vi "Reports.Results TE to Test Result Pre JSON V2.vi"(4 "File Data Objs":T1[](array[typedef]), 5 "Test Result In":T10={"#attributes"={"Version"="MTE_1.0.0"}, "Station"={"Name"="", "PN"="", "SN"="", "Rev"="", "PC Name"="", "Location"="", "HW_Config"={"HW_Item"=[]}, "SW_Config"={"SW_Item"=[]}}, "Test Run"={"Operator"="", "Start Time"=timestamp(0 s since 1904-01-01), "Duration(s)"=0.0, "Mode"="", "Comment"="", "ProcessStep"=""}, "Test Sequence"={"Name"="", "Config"={"Config_Item"=[]}}, "UUTs"={"UUT"=[]}} {"UUTs"."UUT"."Measurements"."Measurement"."Status" items=["LOG", "PASS", "FAIL", "ERROR"]}) -> (1 "Test Result V2":T2={"Type"="Test Data", "Version"="1.0.0", "TestEvent"={"ProcessStep"="", "StartTime"="", "EndTime"="", "Mode"="", "Operator"="", "Comment"="", "Result"={"State"="", "Code"=0, "Desc"="", "Details"=""}}, "UUTInfo"={"Product"="", "Description"="", "PN"="", "SN"="", "LotNumber"="", "DateCode"="", "AltID"="", "Revision"="", "Properties"=[]}, "Station"={"Name"="", "Location"="", "ConfigID"="", "PCName"="", "Slot"=""}, "TestSequence"={"Name"="", "Setup"=[]}, "ResultData"=[], "DataObjs"=[]})   [LabVIEW 2018]
uses:
  Results/Result XML/TestResult.FullResultData.ctl
  Results/Result XML/TestResult.Station Info.ctl
  Results/Result XML/TestResult.HW Item.ctl
  Results/Result XML/TestResult.SW Item.ctl
  Results/Result XML/TestResult.Test Run Info.ctl
  Results/Result XML/TestResult.Test Info.ctl
  Results/Result XML/TestResult.UUT Result.ctl
  Results/Result XML/TestResult.Symptom.ctl
  Results/Result XML/TestResult.Symptom.State.ctl
  Results/Result.Measurement Item.ctl
  Results/Result.Measurement and Attribute Item Status.ctl
  Results/Result XML/TestResult.UUTInfo.ctl
  Report.Result Data JSON V2.0.0.ctl
  Report.Result Test Event.ctl
  Report.Result State.ctl
  Report.Result UUTInfo.ctl
  Report.Result Test Station.ctl
  Report.Result Test Sequence.ctl
  Report.Result Measurement JSON Safe.ctl
  Report.Result DataObject.ctl
  Report.Result FileDataObject.ctl
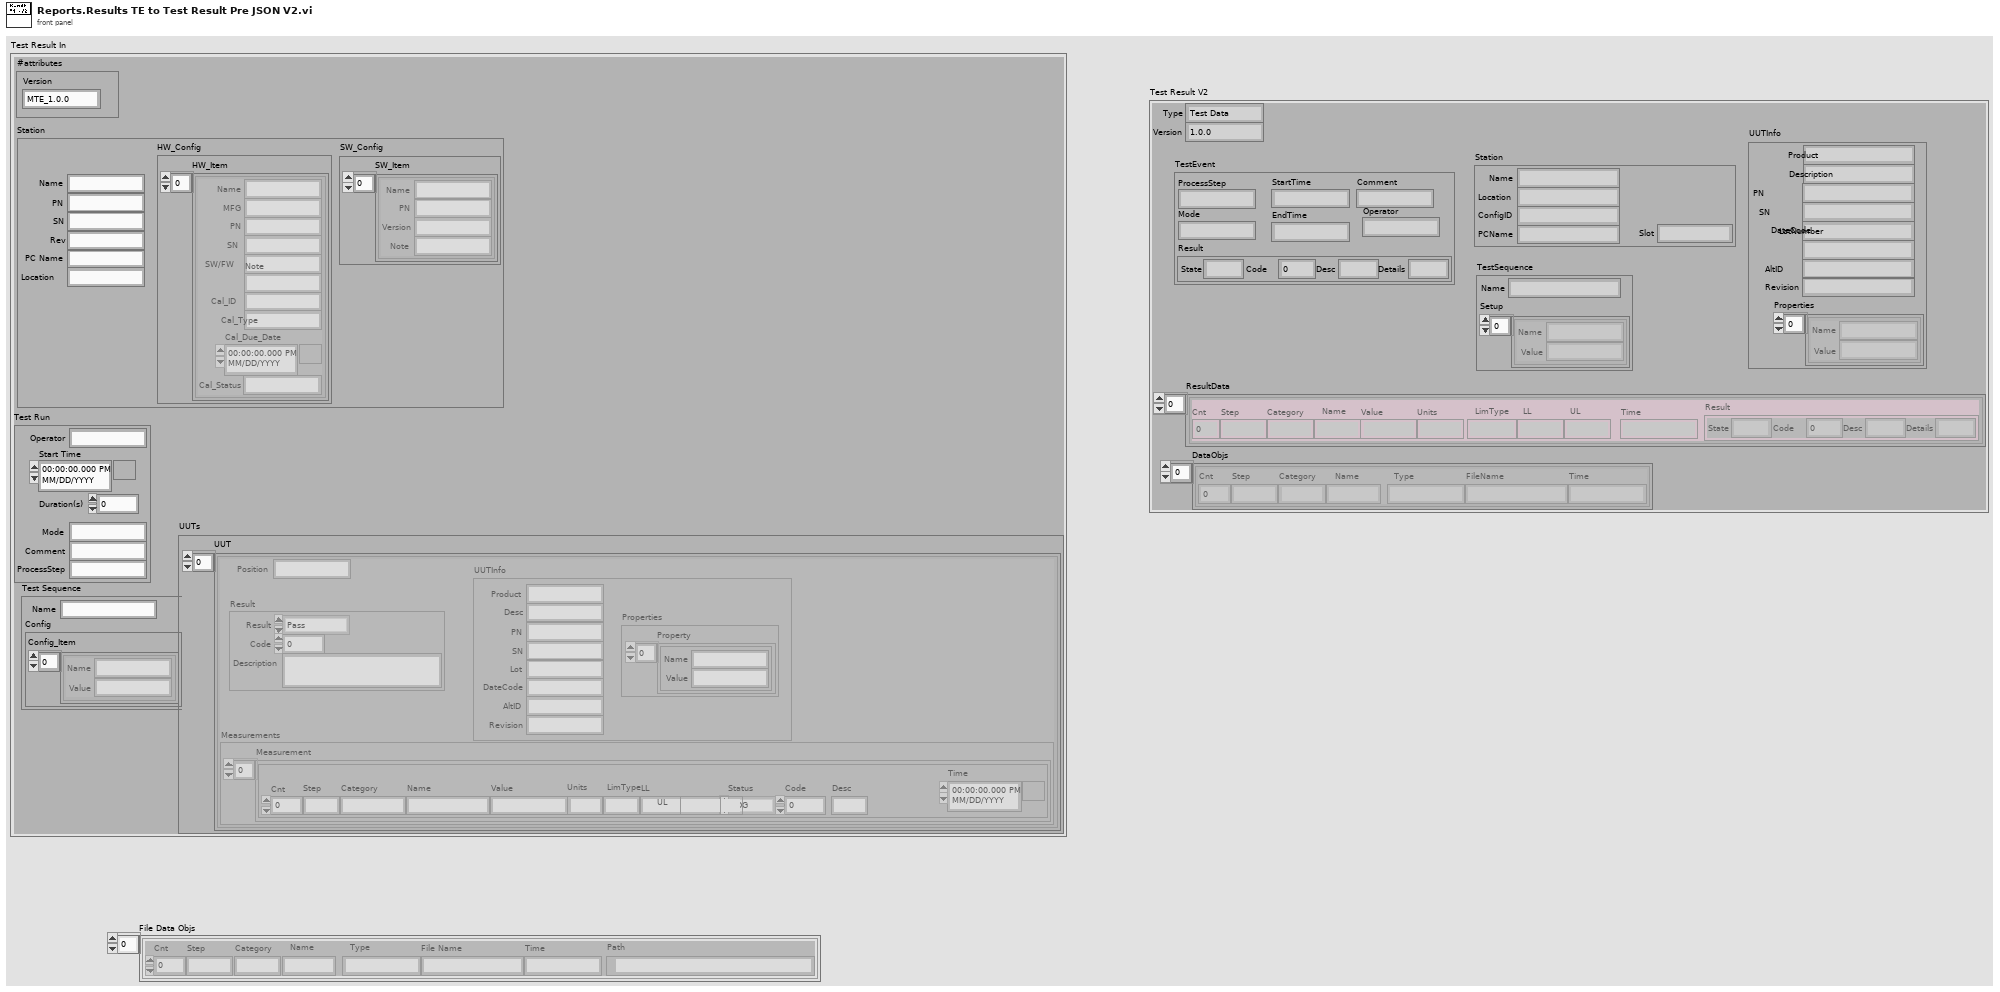
[diagram p1: front panel]
types:
  T1 = typedef "Report.Result FileDataObject.ctl" = cluster{"Cnt":i32, "Step":string, "Category":string, "Name":string, "Type":string, "File Name":string, "Time":string, "Path":path}
  T2 = typedef "Report.Result Data JSON V2.0.0.ctl" = cluster{"Type":string, "Version":string, "TestEvent":T3, "UUTInfo":T5, "Station":T6, "TestSequence":T7, "ResultData":T8[], "DataObjs":T9[]}
  T3 = typedef "Report.Result Test Event.ctl" = cluster{"ProcessStep":string, "StartTime":string, "EndTime":string, "Mode":string, "Operator":string, "Comment":string, "Result":T4}
  T4 = typedef "Report.Result State.ctl" = cluster{"State":string, "Code":i32, "Desc":string, "Details":string}
  T5 = typedef "Report.Result UUTInfo.ctl" = cluster{"Product":string, "Description":string, "PN":string, "SN":string, "LotNumber":string, "DateCode":string, "AltID":string, "Revision":string, "Properties":cluster{"Name":string, "Value":string}[]}
  T6 = typedef "Report.Result Test Station.ctl" = cluster{"Name":string, "Location":string, "ConfigID":string, "PCName":string, "Slot":string}
  T7 = typedef "Report.Result Test Sequence.ctl" = cluster{"Name":string, "Setup":cluster{"Name":string, "Value":string}[]}
  T8 = typedef "Report.Result Measurement JSON Safe.ctl" = cluster{"Cnt":i32, "Step":string, "Category":string, "Name":string, "Value":string, "Units":string, "LimType":string, "LL":string, "UL":string, "Time":string, "Result":T4}
  T9 = typedef "Report.Result DataObject.ctl" = cluster{"Cnt":i32, "Step":string, "Category":string, "Name":string, "Type":string, "FileName":string, "Time":string}
  T10 = typedef "TestResult.FullResultData.ctl" = cluster{"#attributes":cluster{"Version":string}, "Station":T11, "Test Run":T14, "Test Sequence":T15, "UUTs":cluster{"UUT":T16[]}}
  T11 = typedef "TestResult.Station Info.ctl" = cluster{"Name":string, "PN":string, "SN":string, "Rev":string, "PC Name":string, "Location":string, "HW_Config":cluster{"HW_Item":T12[]}, "SW_Config":cluster{"SW_Item":T13[]}}
  T12 = typedef "TestResult.HW Item.ctl" = cluster{"Name":string, "MFG":string, "PN":string, "SN":string, "SW/FW":string, "Note":string, "Cal_ID":string, "Cal_Type":string, "Cal_Due_Date":timestamp, "Cal_Status":string}
  T13 = typedef "TestResult.SW Item.ctl" = cluster{"Name":string, "PN":string, "Version":string, "Note":string}
  T14 = typedef "TestResult.Test Run Info.ctl" = cluster{"Operator":string, "Start Time":timestamp, "Duration(s)":dbl, "Mode":string, "Comment":string, "ProcessStep":string}
  T15 = typedef "TestResult.Test Info.ctl" = cluster{"Name":string, "Config":cluster{"Config_Item":cluster{"Name":string, "Value":string}[]}}
  T16 = typedef "TestResult.UUT Result.ctl" = cluster{"Position":string, "Result":T17, "Measurements":cluster{"Measurement":T19[]}, "UUTInfo":T21}
  T17 = typedef "TestResult.Symptom.ctl" = cluster{"Result":T18, "Code":i32, "Description":string}
  T18 = typedef "TestResult.Symptom.State.ctl" = enum16{"Pass", "Fail", "Error", "Aborted", "Completed", "Logged"}
  T19 = typedef "Result.Measurement Item.ctl" = cluster{"Cnt":i32, "Step":string, "Category":string, "Name":string, "Value":string, "Units":string, "LimType":string, "LL":string, "UL":string, "Status":T20, "Code":i32, "Desc":string, "Time":timestamp}
  T20 = typedef "Result.Measurement and Attribute Item Status.ctl" = i32
  T21 = typedef "TestResult.UUTInfo.ctl" = cluster{"Product":string, "Desc":string, "PN":string, "SN":string, "Lot":string, "DateCode":string, "AltID":string, "Revision":string, "Properties":cluster{"Property":cluster{"Name":string, "Value":string}[]}}
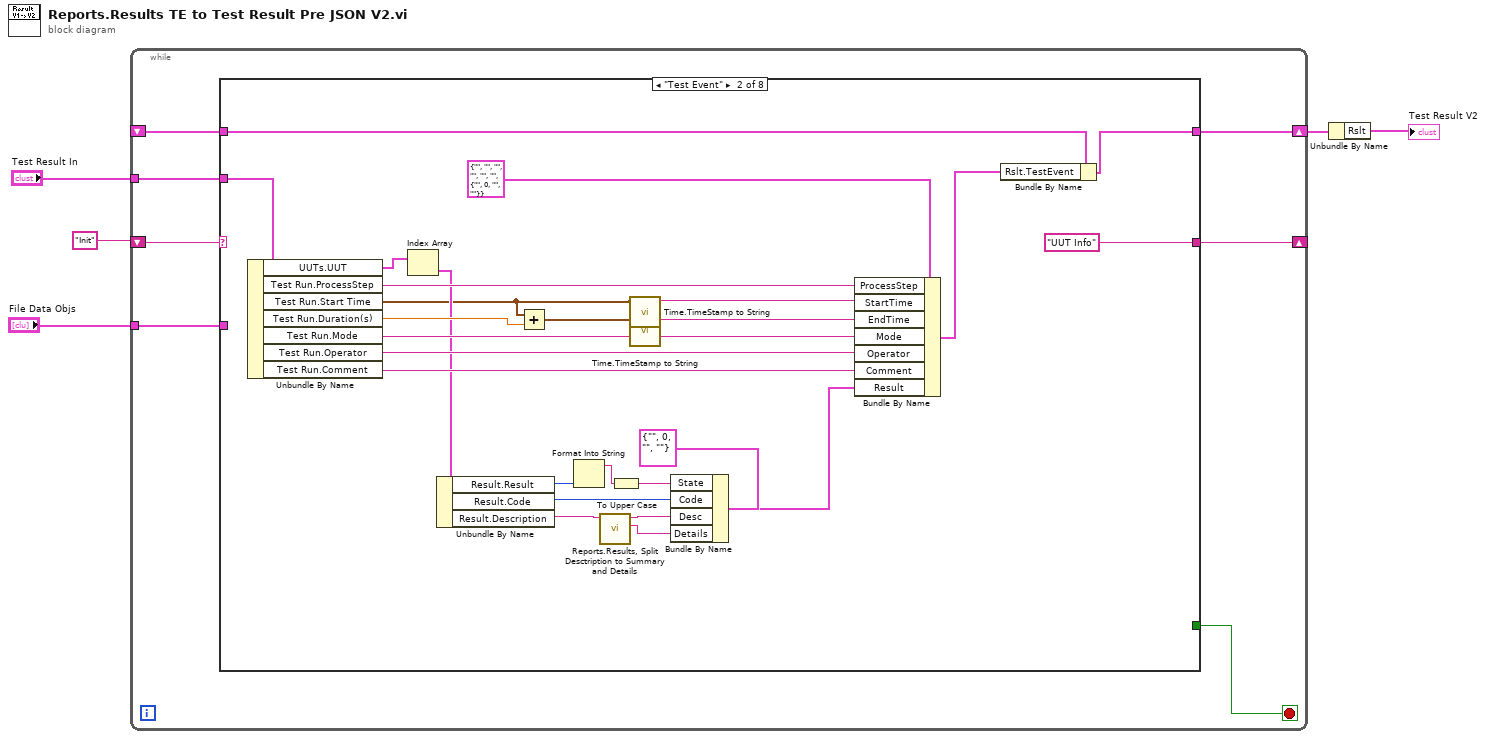
[diagram p0: block diagram]
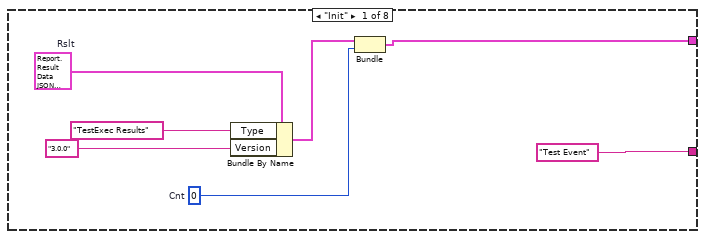
[diagram p2: hidden frame]
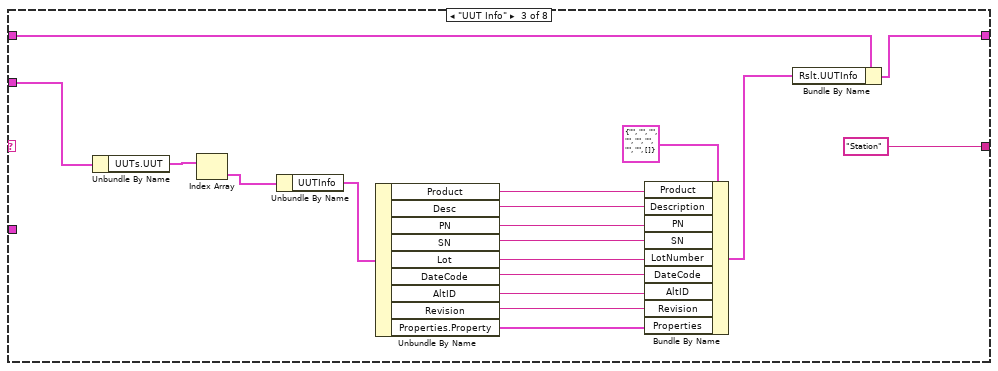
[diagram p3: hidden frame]
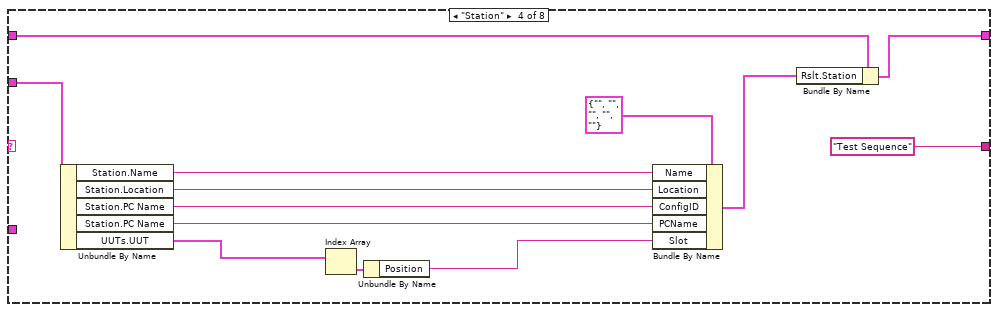
[diagram p4: hidden frame]
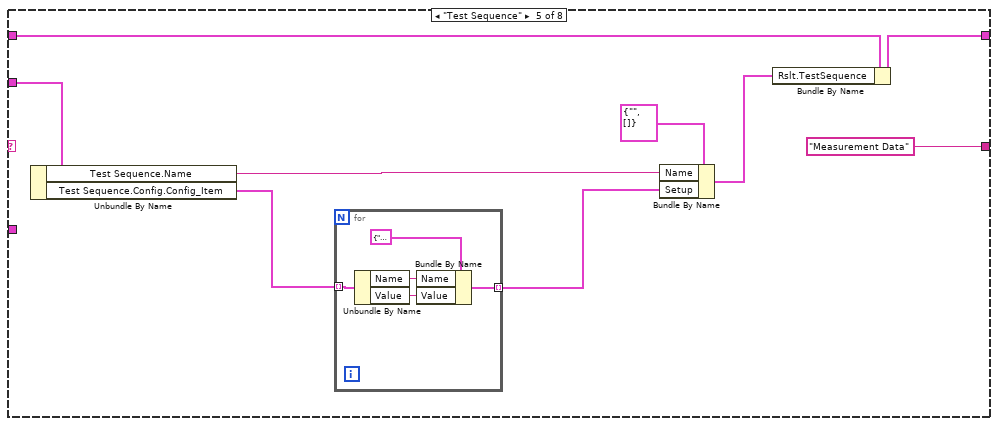
[diagram p5: hidden frame]
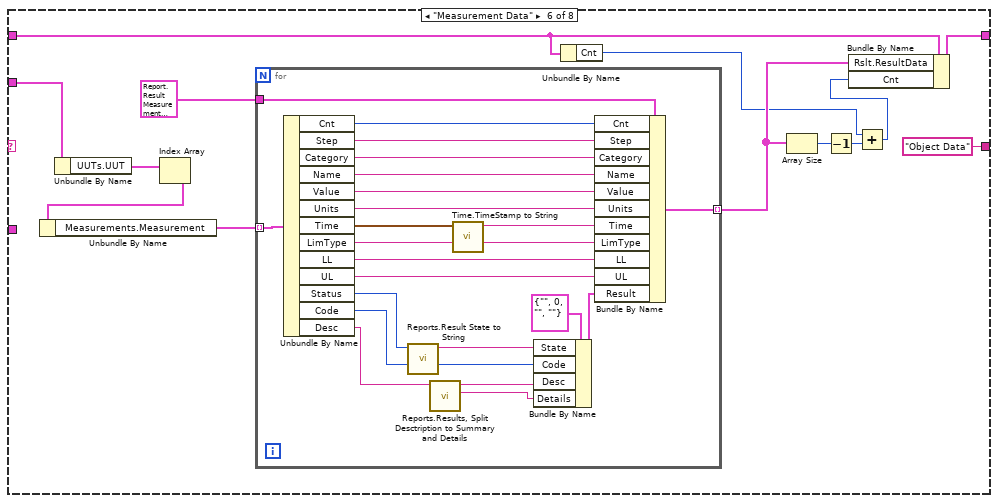
[diagram p6: hidden frame]
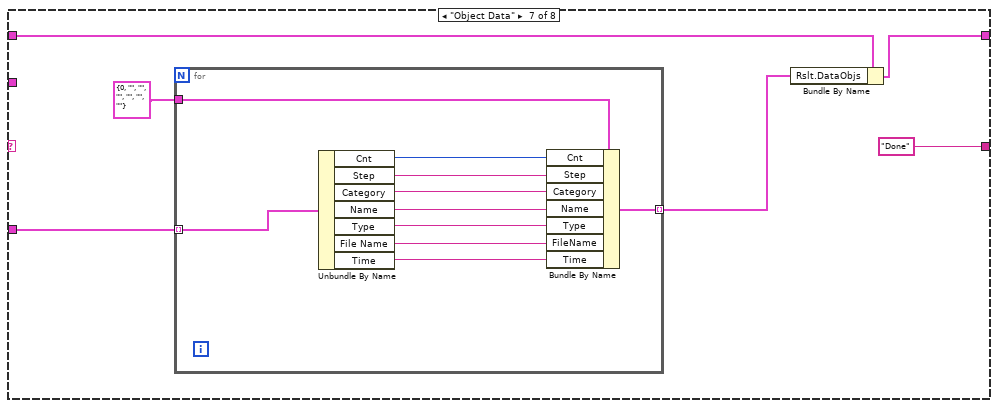
[diagram p7: hidden frame]
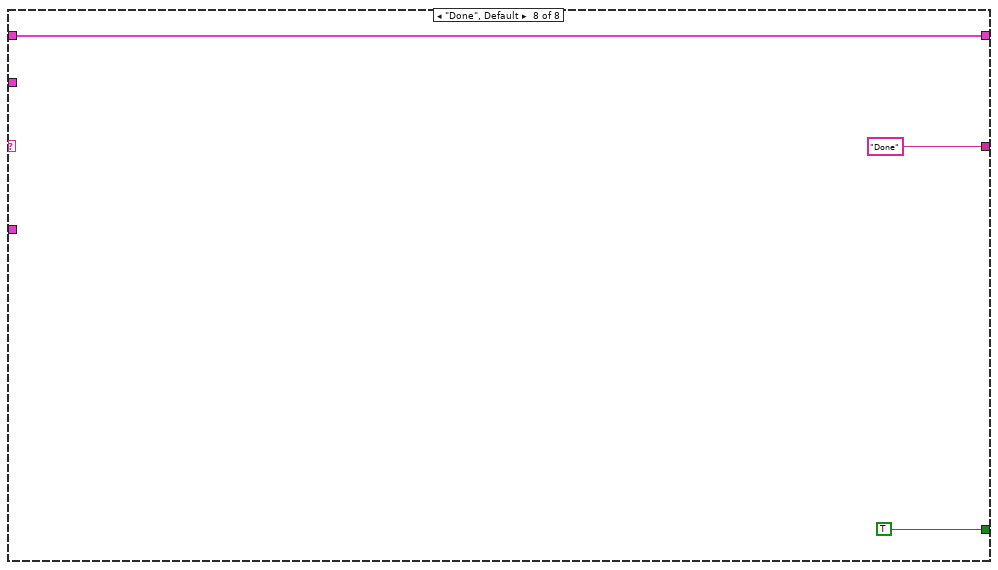
[diagram p8: hidden frame]
diagram:
  n1 = while {
    tunnel: "Test Result In" -> [w12]
    shift-right: [w10] -> w2
    shift-left: _ -> [w11]
    shift-right: [w7] -> _
    shift-left: "Init" -> [w8]
    tunnel: "File Data Objs" -> [w6]
    stop <- w9 stop-if-true
    n2 = case shown="\"Test Event\"" w8 {
      tunnel: w12 -> [_ w39 w59 w72 w81 w102 _ _]
      tunnel: w11 -> [_ w45 w63 w76 w85 w93 w126 w144]
      tunnel: [w14 w44 w62 w75 w84 w103 w131 w144] -> w10
      tunnel: [_ _ _ _ _ _ _ TRUE] -> w9
      tunnel: ["Test Event" ("Version") "UUT Info" ("Version") "Station" ("Version") "Test Sequence" ("Version") "Measurement Data" ("Version") "Object Data" ("Version") "Done" ("Version") "Done"] -> w7
      tunnel: w6 -> [_ _ _ _ _ _ w127 _]
      frame "Init" {
        w13 = 0  # Cnt
        w17 = T2 {"Type"="Test Data", "Version"="1.0.0", "TestEvent"={"ProcessStep"="", "StartTime"="", "EndTime"="", "Mode"="", "Operator"="", "Comment"="", "Result"={"State"="", "Code"=0, "Desc"="", "Details"=""}}, "UUTInfo"={"Product"="", "Description"="", "PN"="", "SN"="", "LotNumber"="", "DateCode"="", "AltID"="", "Revision"="", "Properties"=[]}, "Station"={"Name"="", "Location"="", "ConfigID"="", "PCName"="", "Slot"=""}, "TestSequence"={"Name"="", "Setup"=[]}, "ResultData"=[], "DataObjs"=[]}  # Rslt
        n3 = Bundle By Name(cluster=w17, "Type"="TestExec Results", "Version"="3.0.0") -> (w15:T2)
        n4 = Bundle("Rslt"=w15, "Cnt"=w13) -> (w14:cluster{"Rslt":T2, "Cnt":i32})  [unwired: 1 in]
      }
      frame "Test Event" {
        n5 = Unbundle By Name(w39) -> ("UUTs.UUT"=w38:T16[], "Test Run.ProcessStep"=w37:string, "Test Run.Start Time"=w27:timestamp, "Test Run.Duration(s)"=w35:dbl, "Test Run.Mode"=w36:string, "Test Run.Operator"=w34:string, "Test Run.Comment"=w33:string)
        n6 = Index Array(array=w38) -> (element=w32:T16)  [unwired: 1 in]
        n7 = Unbundle By Name(w32) -> ("Result.Result"=w30:T18, "Result.Code"=w31:i32, "Result.Description"=w22:string)
        n8 = Add(x=w27, y=w35) -> (x+y=w28:timestamp)
        n9 = Format Into String(w30) -> (resulting string=w23:string)  [unwired: 3 in, 1 out]
        n10 = call "Reports.Results, Split Desctription to Summary and Details.vi"("Description"=w22) -> ("Details"=w21:string, "Summary Description"=w20:string)  [unwired: 9 in]
        n11 = To Upper Case(1:w23) -> (0:w24:string)
        n12 = call "Time.TimeStamp to String.vi"("Time Stamp in"=w27) -> ("Time String Out"=w26:string)  [unwired: 10 in]
        n13 = call "Time.TimeStamp to String.vi"("Time Stamp in"=w28) -> ("Time String Out"=w25:string)  [unwired: 10 in]
        n14 = Bundle By Name(cluster=T4 {"State"="", "Code"=0, "Desc"="", "Details"=""} ("Result"), "State"=w24, "Code"=w31, "Desc"=w20, "Details"=w21) -> (w40:T4)
        n15 = Bundle By Name(cluster=T3 {"ProcessStep"="", "StartTime"="", "EndTime"="", "Mode"="", "Operator"="", "Comment"="", "Result"={"State"="", "Code"=0, "Desc"="", "Details"=""}} ("Test Event"), "ProcessStep"=w37, "StartTime"=w26, "EndTime"=w25, "Mode"=w36, "Operator"=w34, "Comment"=w33, "Result"=w40) -> (w42:T3)
        n16 = Bundle By Name(cluster=w45, "Rslt.TestEvent"=w42) -> (w44:cluster{"Rslt":T2, "Cnt":i32})
      }
      frame "UUT Info" {
        n17 = Unbundle By Name(w59) -> ("UUTs.UUT"=w58:T16[])
        n18 = Index Array(array=w58) -> (element=w57:T16)  [unwired: 1 in]
        n19 = Unbundle By Name(w57) -> ("UUTInfo"=w55:T21)
        n20 = Unbundle By Name(w55) -> ("Product"=w54:string, "Desc"=w53:string, "PN"=w52:string, "SN"=w51:string, "Lot"=w50:string, "DateCode"=w49:string, "AltID"=w48:string, "Revision"=w47:string, "Properties.Property"=w46:cluster{"Name":string, "Value":string}[])
        n21 = Bundle By Name(cluster=T5 {"Product"="", "Description"="", "PN"="", "SN"="", "LotNumber"="", "DateCode"="", "AltID"="", "Revision"="", "Properties"=[]} ("UUTInfo"), "Product"=w54, "Description"=w53, "PN"=w52, "SN"=w51, "LotNumber"=w50, "DateCode"=w49, "AltID"=w48, "Revision"=w47, "Properties"=w46) -> (w60:T5)
        n22 = Bundle By Name(cluster=w63, "Rslt.UUTInfo"=w60) -> (w62:cluster{"Rslt":T2, "Cnt":i32})
      }
      frame "Station" {
        n23 = Unbundle By Name(w72) -> ("Station.Name"=w68:string, "Station.Location"=w67:string, "Station.PC Name"=w66:string, "Station.PC Name"=w65:string, "UUTs.UUT"=w64:T16[])
        n24 = Index Array(array=w64) -> (element=w71:T16)  [unwired: 1 in]
        n25 = Unbundle By Name(w71) -> ("Position"=w69:string)
        n26 = Bundle By Name(cluster=T6 {"Name"="", "Location"="", "ConfigID"="", "PCName"="", "Slot"=""} ("Station"), "Name"=w68, "Location"=w67, "ConfigID"=w66, "PCName"=w65, "Slot"=w69) -> (w73:T6)
        n27 = Bundle By Name(cluster=w76, "Rslt.Station"=w73) -> (w75:cluster{"Rslt":T2, "Cnt":i32})
      }
      frame "Test Sequence" {
        n28 = Unbundle By Name(w81) -> ("Test Sequence.Name"=w79:string, "Test Sequence.Config.Config_Item"=w78:cluster{"Name":string, "Value":string}[])
        n29 = for {
          tunnel: w78 -> [w89] mode=indexing
          tunnel: [w86] -> w77 mode=indexing
          n30 = Unbundle By Name(w89) -> ("Name"=w88:string, "Value"=w87:string)
          n31 = Bundle By Name(cluster=cluster{"Name":string, "Value":string} {"Name"="", "Value"=""} ("Setup"), "Name"=w88, "Value"=w87) -> (w86:cluster{"Name":string, "Value":string})
        }
        n32 = Bundle By Name(cluster=T7 {"Name"="", "Setup"=[]} ("TestSequence"), "Name"=w79, "Setup"=w77) -> (w82:T7)
        n33 = Bundle By Name(cluster=w85, "Rslt.TestSequence"=w82) -> (w84:cluster{"Rslt":T2, "Cnt":i32})
      }
      frame "Measurement Data" {
        n34 = Unbundle By Name(w102) -> ("UUTs.UUT"=w100:T16[])
        n35 = Index Array(array=w100) -> (element=w99:T16)  [unwired: 1 in]
        n36 = Unbundle By Name(w99) -> ("Measurements.Measurement"=w98:T19[])
        n37 = for {
          tunnel: w98 -> [w125] mode=indexing
          tunnel: T8 {"Cnt"=0, "Step"="", "Category"="", "Name"="", "Value"="", "Units"="", "LimType"="", "LL"="", "UL"="", "Time"="", "Result"={"State"="", "Code"=0, "Desc"="", "Details"=""}} ("Measurement") -> [w124]
          tunnel: [w115] -> w95 mode=indexing
          n38 = Unbundle By Name(w125) -> ("Cnt"=w123:i32, "Step"=w122:string, "Category"=w121:string, "Name"=w120:string, "Value"=w119:string, "Units"=w110:string, "Time"=w114:timestamp, "LimType"=w109:string, "LL"=w108:string, "UL"=w107:string, "Status"=w112:T20, "Code"=w116:i32, "Desc"=w106:string)
          n39 = call "Reports.Result State to String.vi"("Result State"=w112) -> ("String Out"=w111:string)  [unwired: 6 in]
          n40 = call "Reports.Results, Split Desctription to Summary and Details.vi"("Description"=w106) -> ("Details"=w104:string, "Summary Description"=w105:string)  [unwired: 9 in]
          n41 = call "Time.TimeStamp to String.vi"("Time Stamp in"=w114) -> ("Time String Out"=w113:string)  [unwired: 10 in]
          n42 = Bundle By Name(cluster=T4 {"State"="", "Code"=0, "Desc"="", "Details"=""} ("Result"), "State"=w111, "Code"=w116, "Desc"=w105, "Details"=w104) -> (w117:T4)
          n43 = Bundle By Name(cluster=w124, "Cnt"=w123, "Step"=w122, "Category"=w121, "Name"=w120, "Value"=w119, "Units"=w110, "Time"=w113, "LimType"=w109, "LL"=w108, "UL"=w107, "Result"=w117) -> (w115:T8)
        }
        n44 = Unbundle By Name(w93) -> ("Cnt"=w92:i32)
        n45 = Array Size(array=w95) -> (size(s)=w96:i32)
        n46 = Decrement(x=w96) -> (x-1=w94:i32)
        n47 = Add(x=w92, y=w94) -> (x+y=w91:i32)
        n48 = Bundle By Name(cluster=w93, "Rslt.ResultData"=w95, "Cnt"=w91) -> (w103:cluster{"Rslt":T2, "Cnt":i32})
      }
      frame "Object Data" {
        n49 = for {
          tunnel: w127 -> [w139] mode=indexing
          tunnel: T9 {"Cnt"=0, "Step"="", "Category"="", "Name"="", "Type"="", "FileName"="", "Time"=""} ("Data Object") -> [w141]
          tunnel: [w140] -> w129 mode=indexing
          n50 = Unbundle By Name(w139) -> ("Cnt"=w138:i32, "Step"=w137:string, "Category"=w136:string, "Name"=w135:string, "Type"=w134:string, "File Name"=w133:string, "Time"=w132:string)
          n51 = Bundle By Name(cluster=w141, "Cnt"=w138, "Step"=w137, "Category"=w136, "Name"=w135, "Type"=w134, "FileName"=w133, "Time"=w132) -> (w140:T9)
        }
        n52 = Bundle By Name(cluster=w126, "Rslt.DataObjs"=w129) -> (w131:cluster{"Rslt":T2, "Cnt":i32})
      }
      frame "Done", Default {
      }
    }
  }
  n53 = Unbundle By Name(w2) -> ("Rslt"=→"Test Result V2":T2)
